vi "KB-内环4相位选点 .vi"(11 "内环3D":dbl[][](array[numeric])) -> (0 "数组":dbl[](array[numeric]), 2 "高度差":dbl, 3 "内环平均高度值":dbl, 4 "x-y":dbl)   [LabVIEW 2015]
uses:
  <vilib>/Math Plots/3D Math Plots/3D Surface/3D Surface XCtrl/3D Surface.xctl
  <vilib>/Math Plots/3D Math Plots/3D Surface/3D Surface Datatype/3D Surface Datatype.lvclass
  <vilib>/Math Plots/3D Math Plots/3D Surface/3D Surface Datatype/Public/Plot Helper (Matrix).vi
panel:
  out "结果":dbl[](array[numeric])
  out "子数组":dbl[][](array[numeric])
  in  "内环坏点数据":dbl[][](array[numeric])=array101x102[10302 elements]
  out "大小 2":i32
  out "波形图":dbl[](graph)
  out "反转的数组":dbl[](array[numeric])
  out "Right max":dbl
  out "left max":dbl
  out "bottom max":dbl
  out "Top max":dbl
  out "right":refnum<class "3D Plot Datatype.lvclass">[](xcontrol) caption="Right"
  out "left":refnum<class "3D Plot Datatype.lvclass">[](xcontrol)
  out "bottom":refnum<class "3D Plot Datatype.lvclass">[](xcontrol)
  out "Top":refnum<class "3D Plot Datatype.lvclass">[](xcontrol)
  out "x":dbl
  out "x/y":dbl[](array[numeric])
  out "大小":i32[](array[numeric])
  out "外环":refnum<class "3D Plot Datatype.lvclass">[](xcontrol)
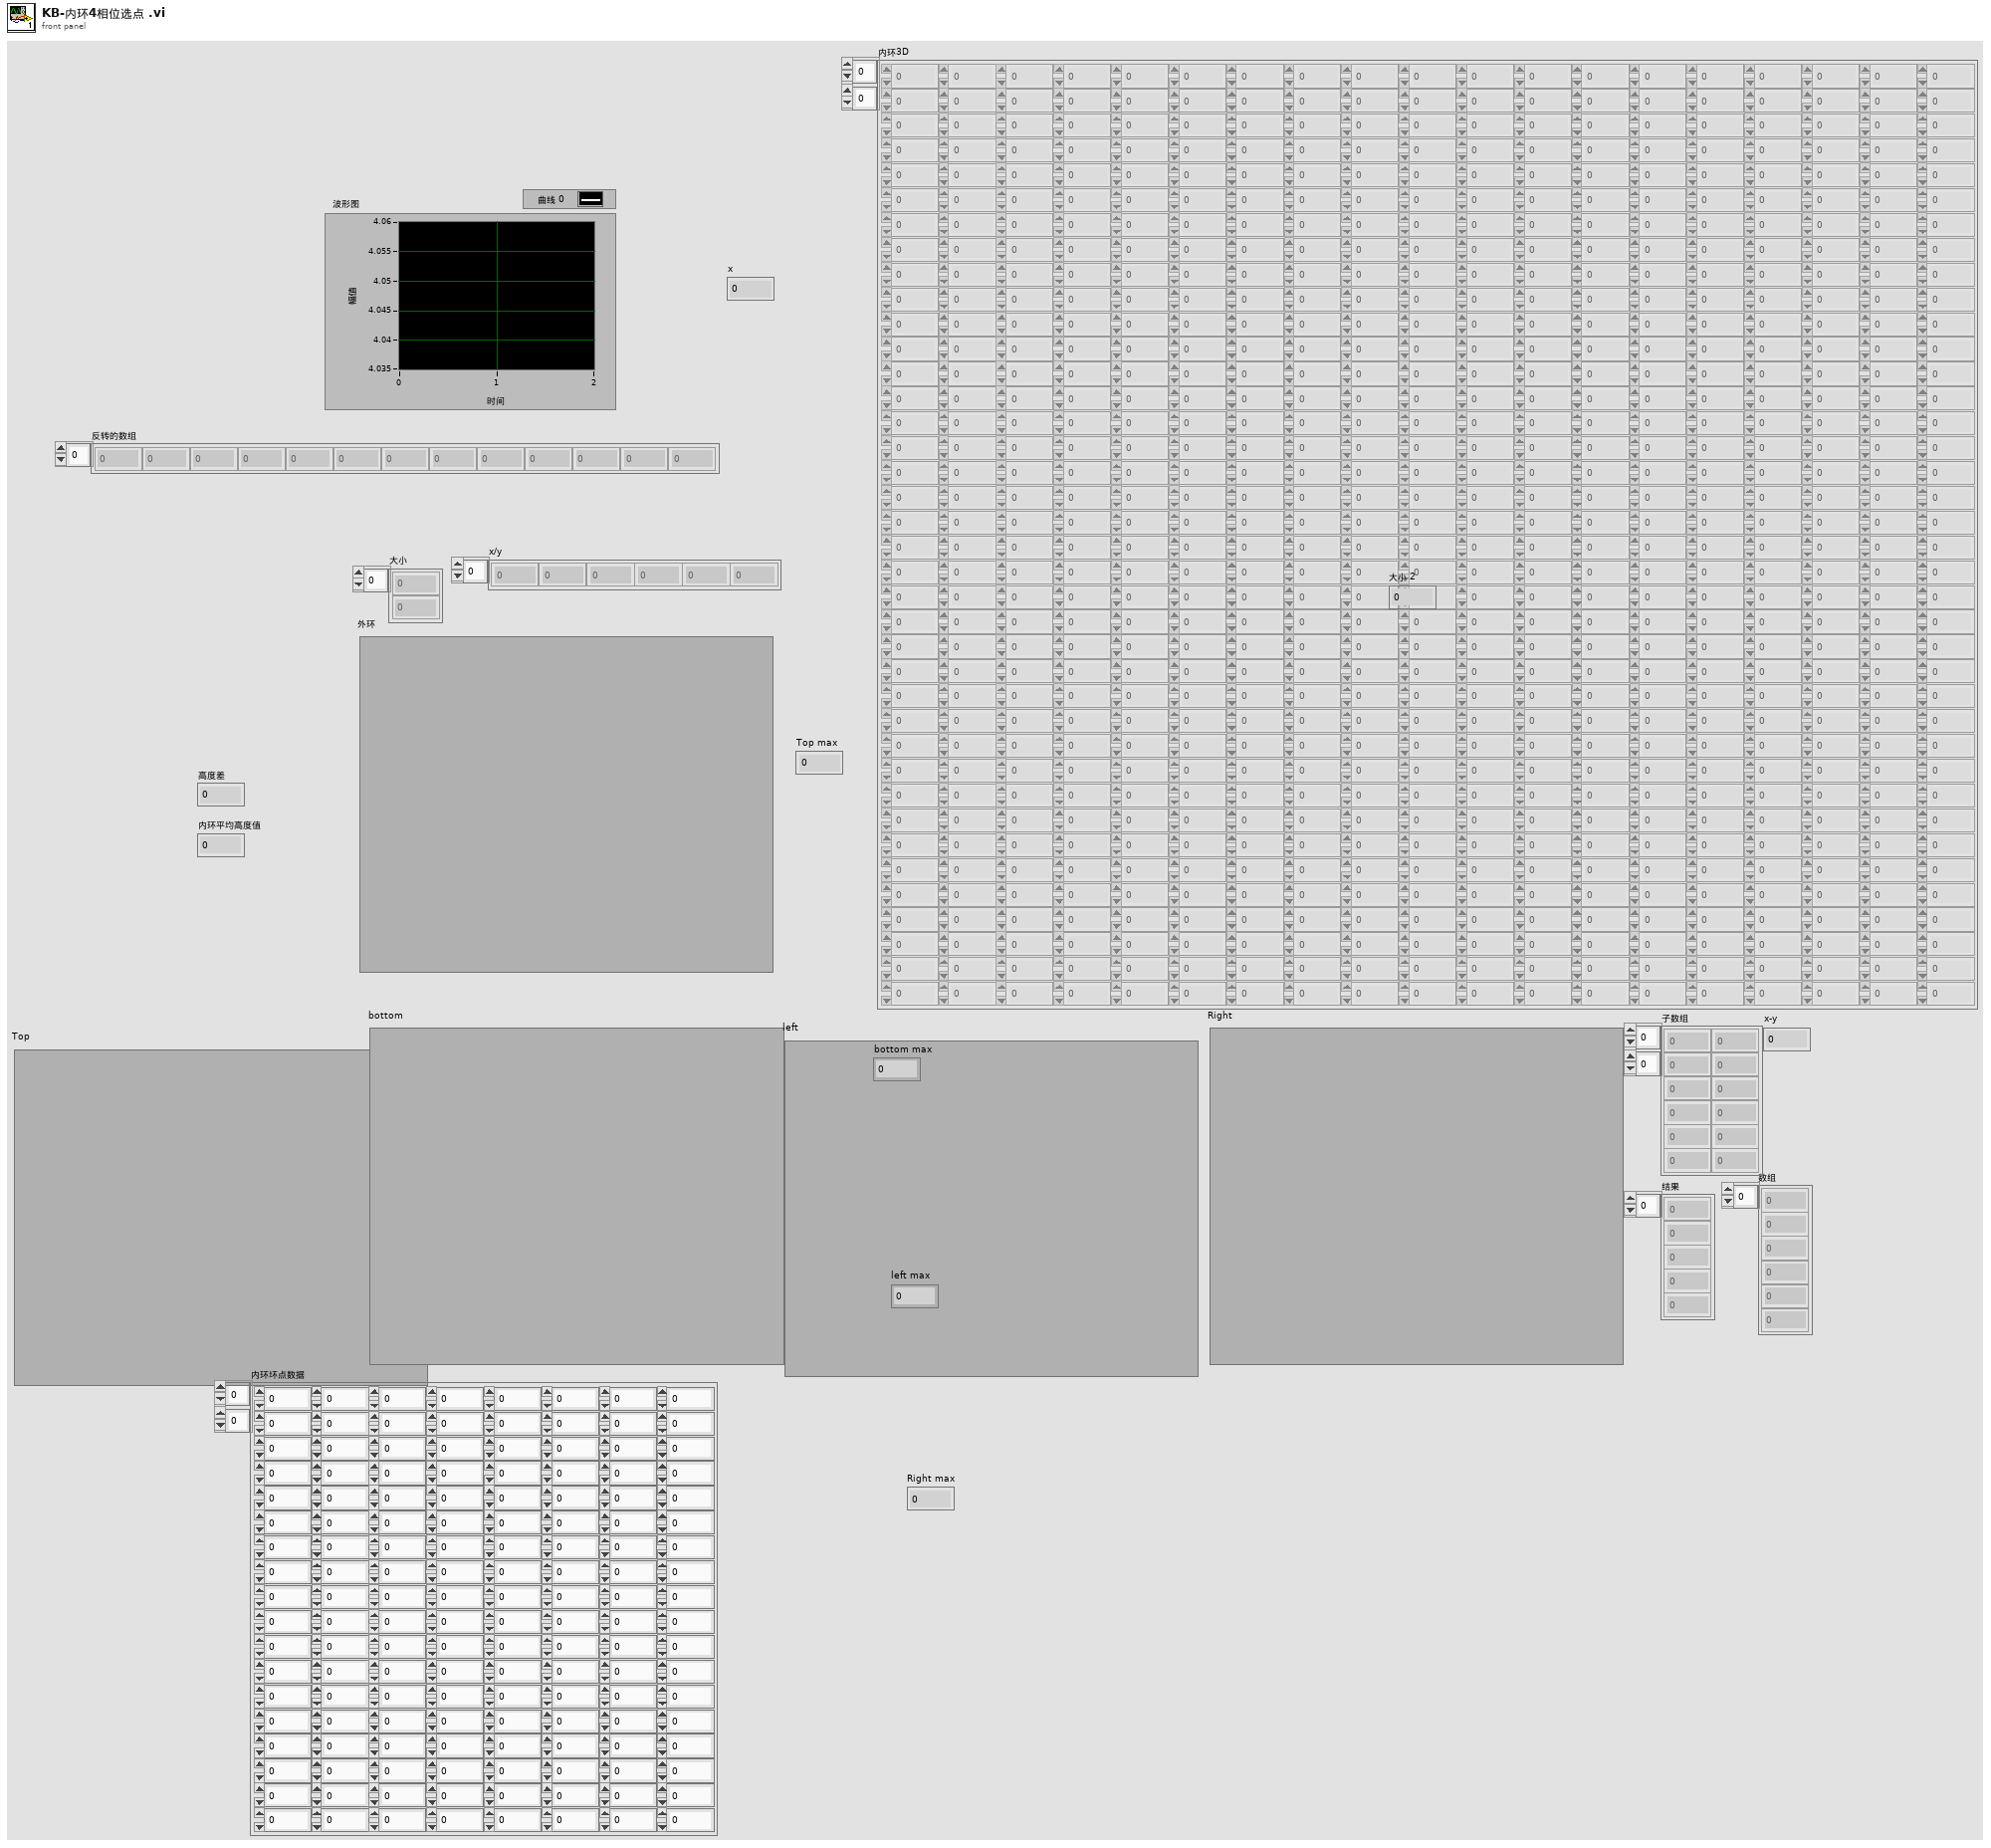
[diagram p1: front panel]
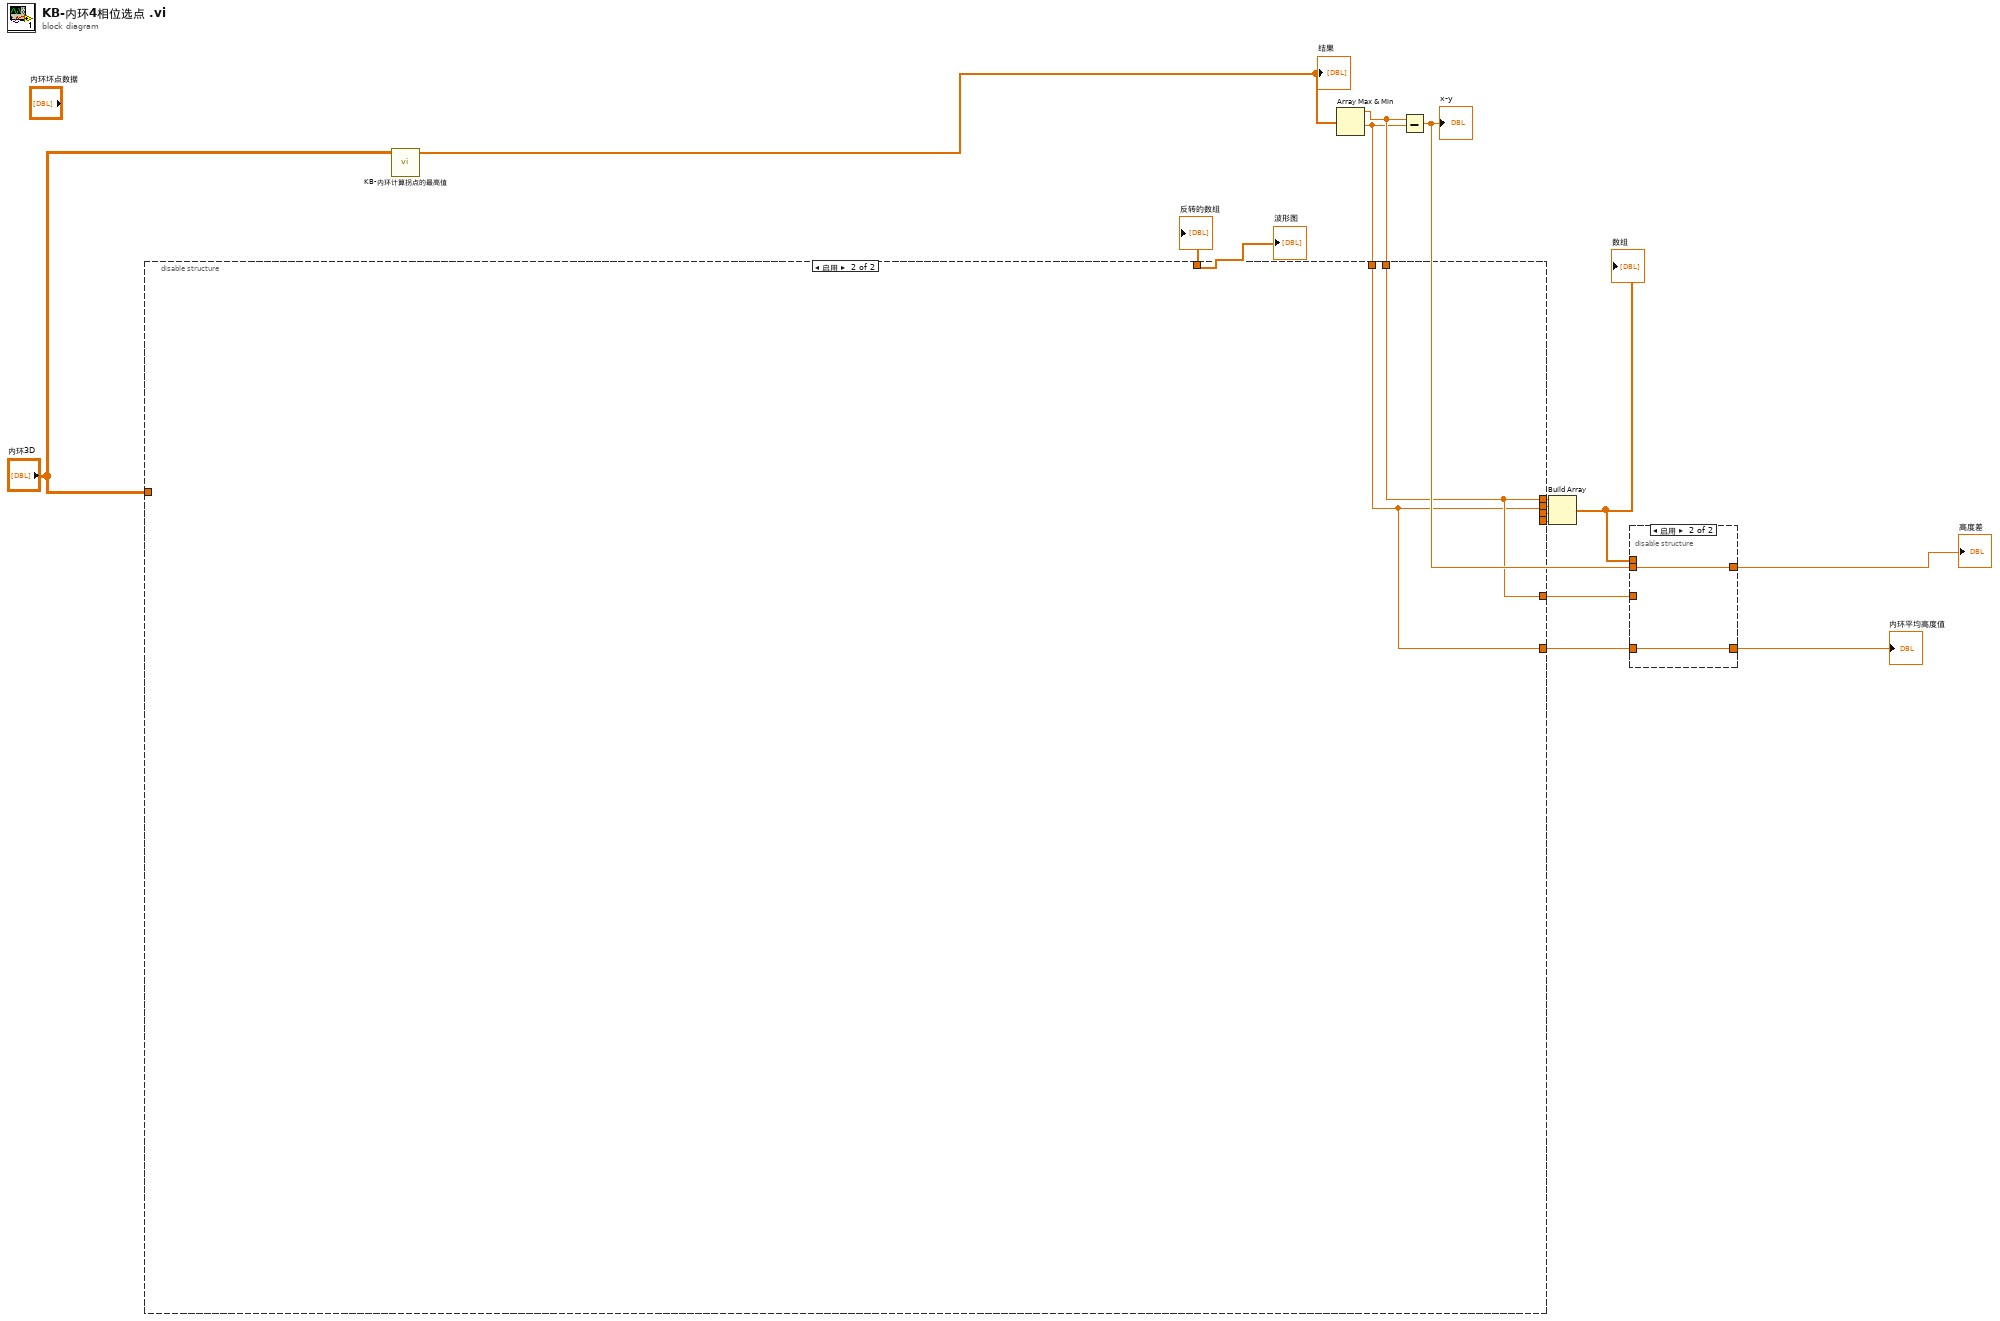
[diagram p0: block diagram]
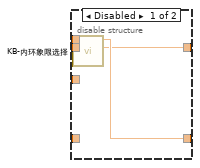
[diagram p2: hidden frame]
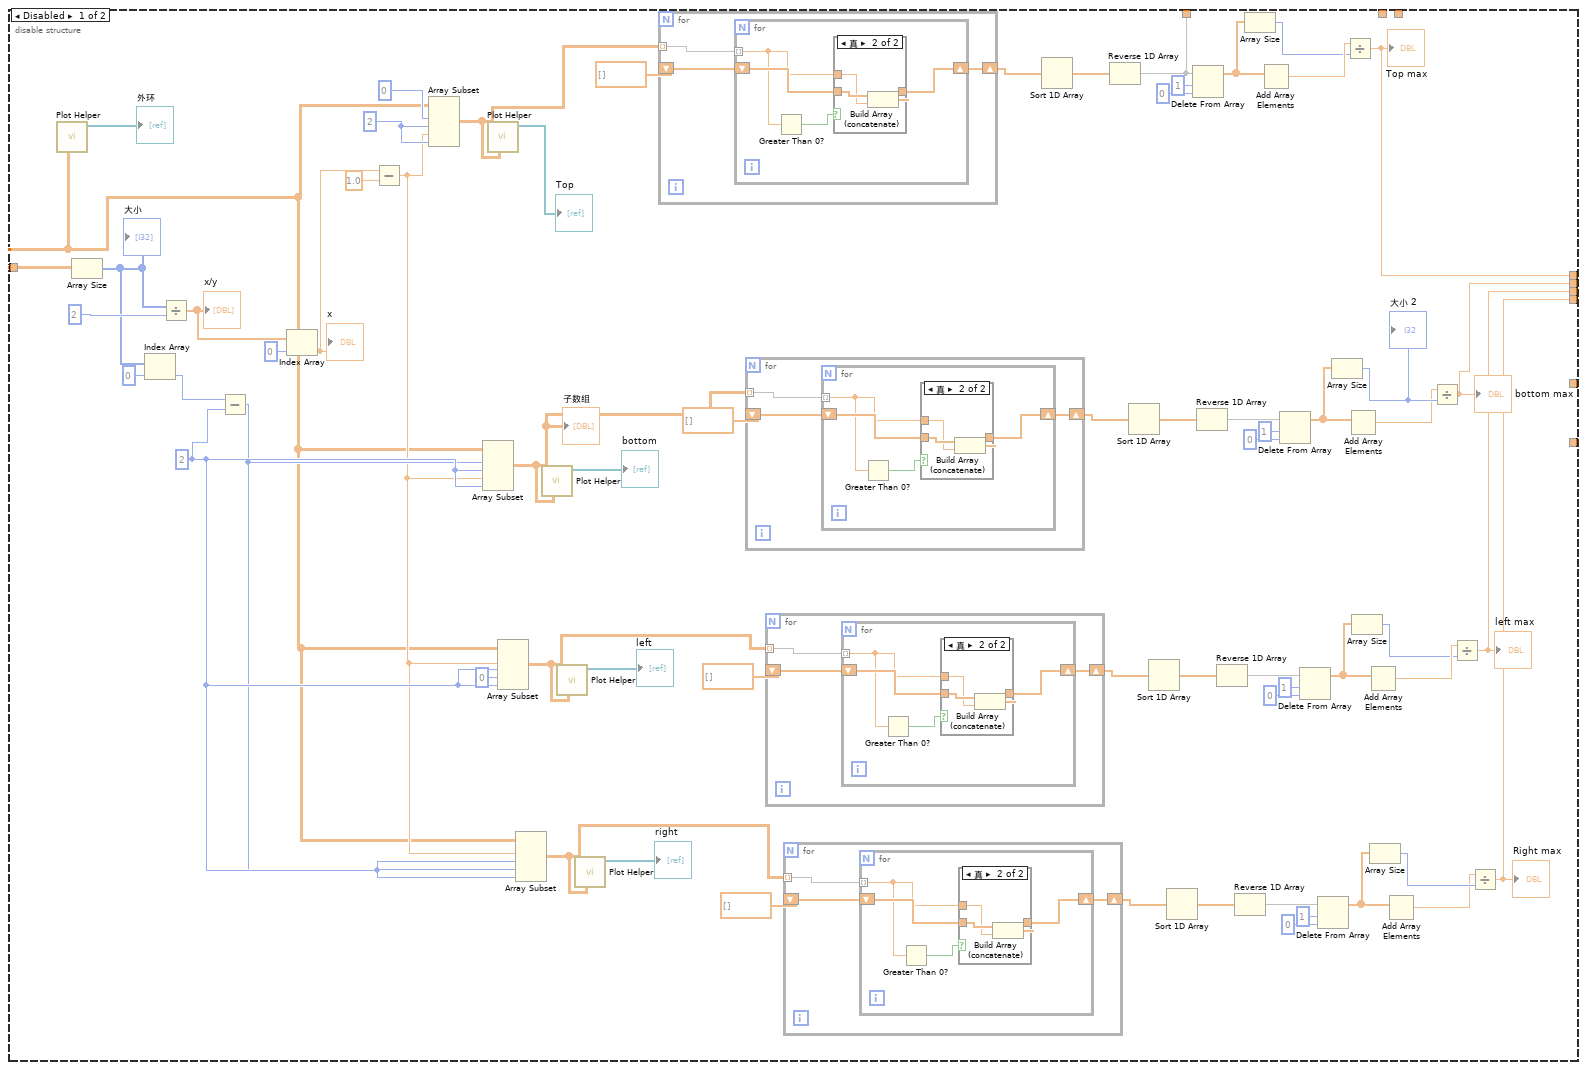
[diagram p3: hidden frame]
diagram:
  n1 = call "KB-内环计算拐点的最高值.vi"("二维内环数组"="内环3D") -> ("结果"=w6:dbl[])  [unwired: 10 in]
  "结果" <- w6
  n2 = Array Max & Min(array=w6) -> (max value=w5:dbl, min value=w4:dbl)  [unwired: 2 out]
  n3 = disable-structure shown="启用" {
    disable-tunnel: [w21 w125] -> w15
    disable-tunnel: [w20 w124] -> w14
    disable-tunnel: [w19 _] -> w13
    disable-tunnel: [w18 _] -> w12
    disable-tunnel: [w17 _] -> w11
    disable-tunnel: "内环3D" -> [w16 _]
    disable-tunnel: w5 -> [_ w125]
    disable-tunnel: w4 -> [_ w124]
    disable-tunnel: [_ w125] -> w3
    disable-tunnel: [_ w124] -> w1
    frame Disabled {
      w62 = 2 ("长度")
      w74 = 2 ("长度")
      n4 = call-poly <vilib>:"Plot Helper.vi"("z matrix"=w16) -> ("3D Plot lvclass Array out"=→"外环":refnum<class "3D Plot Datatype.lvclass">[])  [unwired: 5 in, 5 out]
      n5 = Array Size(array=w16) -> (size(s)=w68:i32[])
      "大小" <- w68
      n6 = Index Array(array=w68, index=0 ("索引")) -> (element=w66:i32)
      n7 = Divide(x=w68, y=2) -> (x/y=w76:dbl[])
      "x/y" <- w76
      n8 = Subtract(x=w66, y=w62) -> (x-y=w61:i32)
      n9 = Index Array(array=w76, index=0 ("索引")) -> (element=w73:dbl)
      "x" <- w73
      n10 = Subtract(x=w73, y=1.0) -> (x-y=w60:dbl)
      n11 = Array Subset(array=w16, index (row)=0 ("索引"), length (row)=w74, index (col)=w60, length (col)=w74) -> (w59:dbl[][])
      n12 = Array Subset(array=w16, index (row)=w61, length (row)=w62, index (col)=w60, length (col)=w62) -> (w42:dbl[][])
      "子数组" <- w42
      n13 = call-poly <vilib>:"Plot Helper.vi"("z matrix"=w59) -> ("3D Plot lvclass Array out"=→"Top":refnum<class "3D Plot Datatype.lvclass">[])  [unwired: 5 in, 5 out]
      n14 = Array Subset(array=w16, index (row)=w60, length (row)=w62, index (col)=0 ("索引"), length (col)=w62) -> (w32:dbl[][])
      n15 = Array Subset(array=w16, index (row)=w60, length (row)=w62, index (col)=w61, length (col)=w62) -> (w22:dbl[][])
      n16 = call-poly <vilib>:"Plot Helper.vi"("z matrix"=w42) -> ("3D Plot lvclass Array out"=→"bottom":refnum<class "3D Plot Datatype.lvclass">[])  [unwired: 5 in, 5 out]
      n17 = call-poly <vilib>:"Plot Helper.vi"("z matrix"=w32) -> ("3D Plot lvclass Array out"=→"left":refnum<class "3D Plot Datatype.lvclass">[])  [unwired: 5 in, 5 out]
      n18 = call-poly <vilib>:"Plot Helper.vi"("z matrix"=w22) -> ("3D Plot lvclass Array out"=→"right":refnum<class "3D Plot Datatype.lvclass">[])  [unwired: 5 in, 5 out]
      n19 = for {
        shift-right: [w113] -> w58
        shift-left: dbl[] [] -> [w115]
        tunnel: w59 -> [w114] mode=indexing
        n20 = for {
          tunnel: w114 -> [w117] mode=indexing
          shift-right: [w118] -> w113
          shift-left: w115 -> [w119]
          n21 = Greater Than 0?(x=w117) -> (x > 0?=w116:bool)
          n22 = case shown="真" w116 {
            tunnel: w119 -> [w120 w123]
            tunnel: w117 -> [_ w122]
            tunnel: [w120 w121] -> w118
            frame False {
            }
            frame True {
              n23 = Build Array (concatenate)(w123, w122) -> (w121:dbl[])
            }
          }
        }
      }
      n24 = for {
        shift-right: [w102] -> w44
        shift-left: dbl[] [] -> [w104]
        tunnel: w42 -> [w103] mode=indexing
        n25 = for {
          tunnel: w103 -> [w106] mode=indexing
          shift-right: [w107] -> w102
          shift-left: w104 -> [w108]
          n26 = Greater Than 0?(x=w106) -> (x > 0?=w105:bool)
          n27 = case shown="真" w105 {
            tunnel: w108 -> [w109 w112]
            tunnel: w106 -> [_ w111]
            tunnel: [w109 w110] -> w107
            frame False {
            }
            frame True {
              n28 = Build Array (concatenate)(w112, w111) -> (w110:dbl[])
            }
          }
        }
      }
      n29 = for {
        shift-right: [w91] -> w40
        shift-left: dbl[] [] -> [w93]
        tunnel: w32 -> [w92] mode=indexing
        n30 = for {
          tunnel: w92 -> [w95] mode=indexing
          shift-right: [w96] -> w91
          shift-left: w93 -> [w97]
          n31 = Greater Than 0?(x=w95) -> (x > 0?=w94:bool)
          n32 = case shown="真" w94 {
            tunnel: w97 -> [w98 w101]
            tunnel: w95 -> [_ w100]
            tunnel: [w98 w99] -> w96
            frame False {
            }
            frame True {
              n33 = Build Array (concatenate)(w101, w100) -> (w99:dbl[])
            }
          }
        }
      }
      n34 = for {
        shift-right: [w80] -> w24
        shift-left: dbl[] [] -> [w82]
        tunnel: w22 -> [w81] mode=indexing
        n35 = for {
          tunnel: w81 -> [w84] mode=indexing
          shift-right: [w85] -> w80
          shift-left: w82 -> [w86]
          n36 = Greater Than 0?(x=w84) -> (x > 0?=w83:bool)
          n37 = case shown="真" w83 {
            tunnel: w86 -> [w87 w90]
            tunnel: w84 -> [_ w89]
            tunnel: [w87 w88] -> w85
            frame False {
            }
            frame True {
              n38 = Build Array (concatenate)(w90, w89) -> (w88:dbl[])
            }
          }
        }
      }
      n39 = Sort 1D Array(array=w58) -> (sorted array=w52:dbl[])
      n40 = Reverse 1D Array(array=w52) -> (reversed array=w17:dbl[])
      n41 = Sort 1D Array(array=w44) -> (sorted array=w51:dbl[])
      n42 = Sort 1D Array(array=w40) -> (sorted array=w33:dbl[])
      n43 = Sort 1D Array(array=w24) -> (sorted array=w31:dbl[])
      n44 = Delete From Array(array=w17, length=1 ("长度"), index=0 ("索引")) -> (array with subset deleted=w55:dbl[])  [unwired: 1 out]
      n45 = Reverse 1D Array(array=w51) -> (reversed array=w46:dbl[])
      n46 = Reverse 1D Array(array=w33) -> (reversed array=w38:dbl[])
      n47 = Reverse 1D Array(array=w31) -> (reversed array=w26:dbl[])
      n48 = Array Size(array=w55) -> (size(s)=w53:i32)
      n49 = Add Array Elements(numeric array=w55) -> (sum=w54:dbl)
      n50 = Delete From Array(array=w46, length=1 ("长度"), index=0 ("索引")) -> (array with subset deleted=w48:dbl[])  [unwired: 1 out]
      n51 = Delete From Array(array=w38, length=1 ("长度"), index=0 ("索引")) -> (array with subset deleted=w36:dbl[])  [unwired: 1 out]
      n52 = Delete From Array(array=w26, length=1 ("长度"), index=0 ("索引")) -> (array with subset deleted=w28:dbl[])  [unwired: 1 out]
      n53 = Array Size(array=w48) -> (size(s)=w50:i32)
      "大小 2" <- w50
      n54 = Divide(x=w54, y=w53) -> (x/y=w21:dbl)
      "Top max" <- w21
      n55 = Add Array Elements(numeric array=w48) -> (sum=w49:dbl)
      n56 = Array Size(array=w36) -> (size(s)=w34:i32)
      n57 = Add Array Elements(numeric array=w36) -> (sum=w35:dbl)
      n58 = Array Size(array=w28) -> (size(s)=w30:i32)
      n59 = Add Array Elements(numeric array=w28) -> (sum=w29:dbl)
      n60 = Divide(x=w49, y=w50) -> (x/y=w20:dbl)
      "bottom max" <- w20
      n61 = Divide(x=w35, y=w34) -> (x/y=w19:dbl)
      "left max" <- w19
      n62 = Divide(x=w29, y=w30) -> (x/y=w18:dbl)
      "Right max" <- w18
    }
    frame Enabled {
    }
  }
  "反转的数组" <- w11
  "波形图" <- w11
  n63 = Subtract(x=w5, y=w4) -> (x-y=w2:dbl)
  "x-y" <- w2
  n64 = Build Array(w15, w14, w13, w12) -> (w10:dbl[])
  "数组" <- w10
  n65 = disable-structure shown="启用" {
    disable-tunnel: w10 -> [w128 _]
    disable-tunnel: [w127 w129] -> w9
    disable-tunnel: [w126 w130] -> w8
    disable-tunnel: w3 -> [_ _]
    disable-tunnel: w2 -> [_ w130]
    disable-tunnel: w1 -> [_ w129]
    frame Disabled {
      n66 = call "KB-内环象限选择.vi"("象限选择"=w128) -> ("内环高度差"=w126:dbl, "内环最高点"=w127:dbl)  [unwired: 9 in]
    }
    frame Enabled {
    }
  }
  "内环平均高度值" <- w9
  "高度差" <- w8
